vi "RectsEqualFloat-lv.vi"(1 "B":T1, 2 "A":T1) -> (0 "A == B?":bool)   [LabVIEW 2024, in "SDL3.lvlib" / "Rect.lvlib"]
doc: "<B>LV Implementation</B>\nSince the SDL function is inlined, we can't access in the shared library. So it's a LabVIEW implementation of the feature.\n\n<B>Summary</B>\nDetermine whether two floating point rectangles are equal\n\n<B>Remarks</B>\nRectangles are considered equal if both are not NULL and each of their x, y, width and height match."
uses:
  FRect--cluster.ctl
  Rect.lvlib
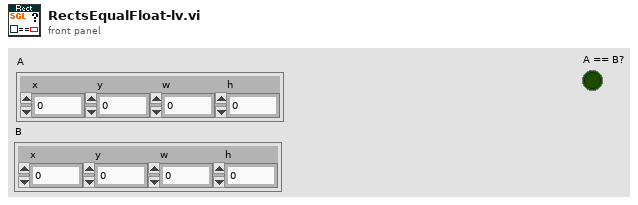
[diagram p1: front panel]
types:
  T1 = typedef "SDL3.lvlib/Rect.lvlib/FRect--cluster.ctl" = cluster{"x":sgl, "y":sgl, "w":sgl, "h":sgl}
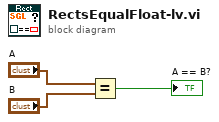
[diagram p0: block diagram]
diagram:
  n1 = Equal?(x="A", y="B") -> (x = y?=→"A == B?":bool)
